vi "32to8.vi"(1 "32data_in":i32 min=-2047 max=2047) -> (0 "8Array":u8[](array[numeric]))   [LabVIEW 2018]
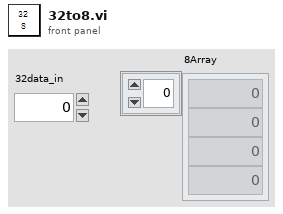
[diagram p1: front panel]
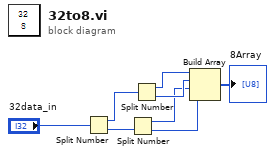
[diagram p0: block diagram]
diagram:
  n1 = Split Number(x="32data_in") -> (hi(x)=w7:u16, lo(x)=w6:u16)
  n2 = Split Number(x=w6) -> (hi(x)=w3:u8, lo(x)=w2:u8)
  n3 = Split Number(x=w7) -> (hi(x)=w5:u8, lo(x)=w4:u8)
  n4 = Build Array(w5, w4, w3, w2) -> (→"8Array":u8[])
